vi "openedWindowsFGV.vi"(7 "Action":enum16{"Get", "Set"}(ring), 8 "error in":errorcluster, 10 "Names in":string[](array[string])) -> (0 "error out":errorcluster, 2 "Names out":string[](array[string]))   [LabVIEW 2023]
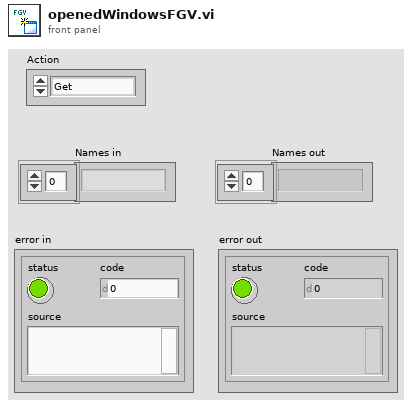
[diagram p1: front panel]
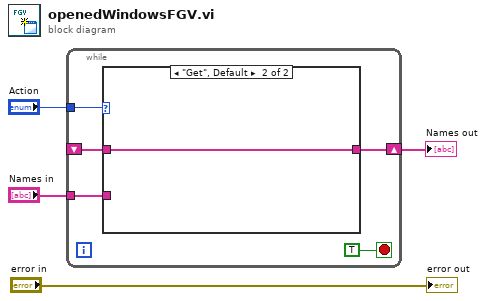
[diagram p0: block diagram]
diagram:
  n1 = while {
    tunnel: "Action" -> [w8]
    tunnel: "Names in" -> [w7]
    shift-right: [w6] -> w2
    shift-left: _ -> [w5]
    stop <- TRUE stop-if-true
    n2 = case shown="\"Get\", Default" w8 {
      tunnel: w7 -> [w10 _]
      tunnel: [w10 w11] -> w6
      tunnel: w5 -> [_ w11]
      frame "Set" {
      }
      frame "Get", Default {
      }
    }
  }
  "Names out" <- w2
  "error out" <- "error in"
